vi "Periodic Tasks.vi"(8 "error in":errorcluster) -> ()   [LabVIEW 2014]
doc: "This VI runs in parallel to other tasks. It can contain as many user-defined periodic loops as you need. These can carry out PID or other sorts of timed response."
uses:
  <vilib>/Rock Robotics/WPI/Solenoid/WPI_SolenoidValue.ctl
  <vilib>/Rock Robotics/WPI/Joystick/WPI_JoystickGetSetRefNum.vi
  <vilib>/Rock Robotics/WPI/RobotDrive/WPI_RobotDriveGetSetRefNum.vi
  <vilib>/Rock Robotics/WPI/Compressor/WPI_CompressorGetSetRefNum.vi
  <vilib>/Rock Robotics/WPI/Ultrasonic/WPI_SonarMB1010DigitalRefNum Registry Get.vi
  Robot Global Data.vi
  <vilib>/Rock Robotics/Network Tables/SD Write Number.vi
  <vilib>/Rock Robotics/WPI/Ultrasonic/WPI_SonarMB1010DigitalGetRange.vi
  <vilib>/Rock Robotics/Network Tables/SD Read Boolean.vi
  <vilib>/Rock Robotics/Network Tables/SD Write Boolean.vi
  <vilib>/Rock Robotics/WPI/Solenoid/WPI_SolenoidSetEnum.vi
  <vilib>/Rock Robotics/Network Tables/SD Write Numeric Array.vi
  <vilib>/addons/control/pid/pid.llb/PID (DBL).vi
  <vilib>/Rock Robotics/Network Tables/SD Write Boolean Array.vi
  <vilib>/addons/control/pid/NI_PID_pid.lvlib
panel:
  in  "Sonar Limit":dbl
  in  "Sonar Offset":dbl
  out "Sonar Distance":dbl=36.82278911564626
  in  "Bypass INI Setting":bool
  in  "step inches":dbl=0.5
  out "Compressor Running":bool
  out "Enabled":bool=TRUE
  out "Manual Winch 2":bool
  in  "Manul drive offset 2":dbl
  in  "Manual scale 2":dbl=2.0 format="%#_13g"
  out "MV: 2":dbl(slide)=2.092346938775512 scale=-100.0..100.0
  out "PV: 2":dbl(slide)=26.0 scale=0.0..100.0
  in  "PID gains 2":T1={"proportional gain (Kc)"=0.6, "integral time (Ti, min)"=0.0, "derivative time (Td, min)"=0.0} {"derivative time (Td, min)" format="%.3f"; "integral time (Ti, min)" format="%.3f"; "proportional gain (Kc)" format="%.3f"}
  in  "output range 2":cluster{"output high":dbl, "output low":dbl}={"output high"=100.0, "output low"=-100.0} {"output low" format="%.2f"; "output high" format="%.2f"}
  out "Process variable and Setpoint 2":cluster{"initial PV":dbl, "SP:":dbl}(graph)={"initial PV"=22.512755102040813, "SP:"=26.0}
  in  "Reset Encoder? 2":bool
  out "Encoder Direction 2":string="Down"
  out "Encoder Distance 2":dbl=22.512755102040813
  in  "Encoder 2 scale":dbl=19.6
  out "In Range? 2":bool=TRUE
  in  "lower limit 2":dbl
  in  "upper limit 2":dbl=100.0
  in  "step inches 2":dbl=0.5
  out "Process variable and Setpoint":cluster{"initial PV":dbl, "SP:":dbl}(graph)={"initial PV"=107.51666666666667, "SP:"=110.0}
  in  "PID gains":T1={"proportional gain (Kc)"=1.0, "integral time (Ti, min)"=0.0, "derivative time (Td, min)"=0.0} {"derivative time (Td, min)" format="%.3f"; "integral time (Ti, min)" format="%.3f"; "proportional gain (Kc)" format="%.3f"}
  out "PV:":dbl(slide)=107.51666666666667 scale=0.0..75.0
  out "SP:":dbl(slide)=110.0 min=0.0 max=0.0 scale=0.0..75.0
  out "MV:":dbl(slide)=2.4833333333333343 scale=-100.0..100.0
  in  "output range":cluster{"output high":dbl, "output low":dbl}={"output high"=5.0, "output low"=-5.0} {"output low" format="%.2f"; "output high" format="%.2f"}
  out "In Range?":bool
  in  "lower limit":dbl
  in  "upper limit":dbl=100.0
  in  "Reset Encoder?":bool
  out "Encoder Direction":string="Down"
  out "Encoder Distance":dbl=107.51666666666667
  in  "Encoder 1 scale":dbl=30.0
  out "Manual Winch 1":bool
  in  "Manul drive offset":dbl
  in  "Manual scale 1":dbl=50.0 format="%#_13g"
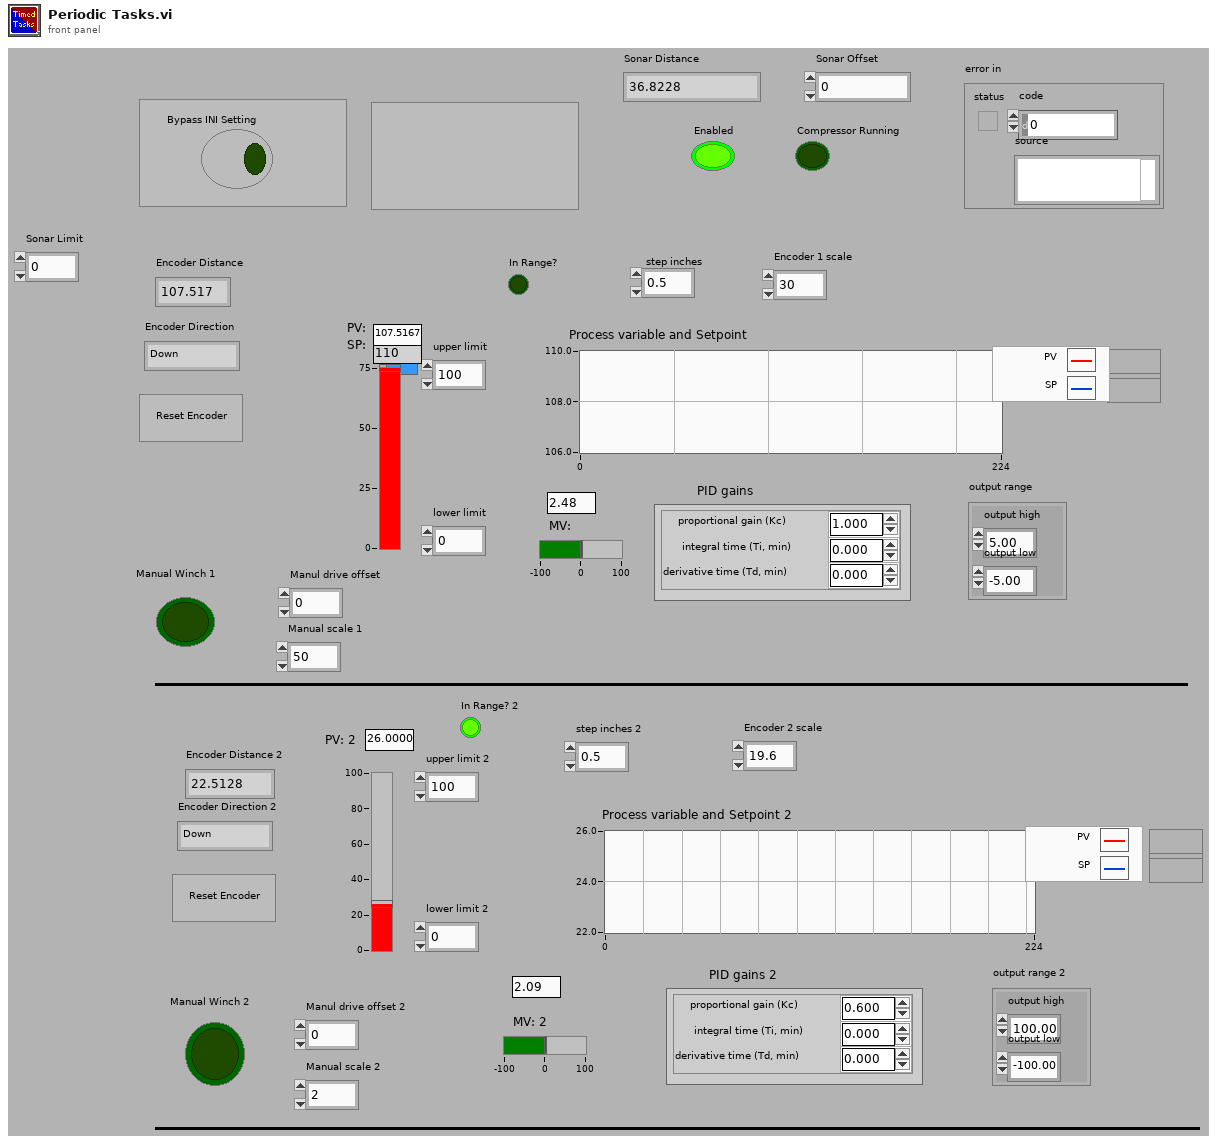
[diagram p1: front panel]
types:
  T1 = cluster{"proportional gain (Kc)":dbl, "integral time (Ti, min)":dbl, "derivative time (Td, min)":dbl}
  T2 = typedef "WPI_MotorControlDeviceRef.ctl" = cluster{"DeviceStatus":errorcluster, "Type":T3, "PWM":cluster{"Controller":T4, "PWM Channel":T5, "DeadBand":T6}, "CAN":cluster{"Device Number":u8, "Control Mode":T7, "Semaphore":T8, "Max Vout":dbl, "TalonSRX Control Mode":T9}, "Invert":bool, "TransformRef":T10, "InvTransformRef":T10}
  T3 = typedef "WPI_MotorControlType.ctl" = enum16{"PWM", "CAN", "CANTalonSRX"}
  T4 = typedef "FPGA_TypedefDigitalModule.ctl" = enum16{"Controller 1"}
  T5 = typedef "FPGA_DIOPWMChannel.ctl" = enum8{"PWM 0", "PWM 1", "PWM 2", "PWM 3", "PWM 4", "PWM 5", "PWM 6", "PWM 7", "PWM 8", "PWM 9", "PWM MXP 0", "PWM MXP 1", "PWM MXP 2", "PWM MXP 3", "PWM MXP 4", "PWM MXP 5", "PWM MXP 6", "PWM MXP 7", "PWM MXP 8", "PWM MXP 9", "Invalid"}
  T6 = typedef "WPI_PWMDeadband.ctl" = cluster{"Name":string, "maxPositivePwm":i32, "minPositivePwm":i32, "centerPwm":i32, "maxNegativePwm":i32, "minNegativePwm":i32, "angularRange":u16}
  T7 = typedef "WPI_CANJaguar_ControlMode.ctl" = enum8{"Percent VBus", "Current", "Speed", "Position", "Voltage"}
  T8 = typedef "Semaphore RefNum" = refnum<k1>
  T9 = typedef "WPI_CANTalonSRX_APIControlMode.ctl" = enum8{"Percent VBus", "Speed", "Position", "Slave", "Unchanged / Invalid"}
  T10 = typedef "WPI_PWMTransform_ConPane.ctl" = refnum<vi>
  T11 = typedef "WPI_JoystickDevRef.ctl" = cluster{"Device":T12}
  T12 = typedef "WPI_JoystickDeviceEnum.ctl" = enum16{"USB 0", "USB 1", "USB 2", "USB 3", "USB 4", "USB 5"}
  T13 = typedef "WPI_RobotDriveDevRef.ctl" = cluster{"DevStatus":errorcluster, "Motors[]":T2[], "Square Inputs":bool, "Max Output":dbl}
  T14 = typedef "WPI_CompressorDevRef.ctl" = cluster{"DevStatus":errorcluster, "Pneumatics Control Module":u8}
  T15 = typedef "WPI_SonarMB1010DigitalDeviceRef.ctl" = cluster{"CounterDevRef":T16, "Scaling factor (s/in)":dbl}
  T16 = typedef "WPI_CounterDevRef.ctl" = cluster{"DevStatus":errorcluster, "CntIndex":T17}
  T17 = typedef "FPGA_CounterCtrSystemIndex.ctl" = enum8{"Ctr 0", "Ctr 1", "Ctr 2", "Ctr 3", "Ctr 4", "Ctr 5", "Ctr 6", "Ctr 7", "Invalid"}
  T18 = typedef "WPI_SwitchDevRef.ctl" = cluster{"DevStatus":errorcluster, "DIO Channel":T19, "Controller":T4, "CntIndex":T17, "Normally Closed":bool}
  T19 = typedef "FPGA_DIOChannel.ctl" = enum8{"DIO 0", "DIO 1", "DIO 2", "DIO 3", "DIO 4", "DIO 5", "DIO 6", "DIO 7", "DIO 8", "DIO 9", "DIO MXP 0", "DIO MXP 1", "DIO MXP 2", "DIO MXP 3", "DIO MXP 4", "DIO MXP 5", "DIO MXP 6", "DIO MXP 7", "DIO MXP 8", "DIO MXP 9", "DIO MXP 10", "DIO MXP 11", "DIO MXP 12", "DIO MXP 13", "DIO MXP 14", "DIO MXP 15", "Invalid"}
  T20 = cluster{"JoystickDevRef":T11, "RobotDriveDevRef":T13}
  T21 = typedef "WPI_EncoderDevRef.ctl" = cluster{"DevStatus":errorcluster, "EncoderIndex":T22, "CounterIndex":T17, "DistancePerCount":dbl, "Decoding Type":T23}
  T22 = typedef "FPGA_EncoderIdx.ctl" = enum8{"Enc 0", "Enc 1", "Enc 2", "Enc 3", "Enc 4", "Enc 5", "Enc 6", "Enc 7", "Invalid"}
  T23 = typedef "WPI_EncoderType.ctl" = enum16{"1x", "2x", "4x"}
  T24 = typedef "WPI_SolenoidDevRef.ctl" = cluster{"DevStatus":errorcluster, "Pneumatics Control Module":u8, "Forward Solenoid Channel":T25, "Reverse Solenoid Channel":T25}
  T25 = typedef "WPI_SolenoidChannel.ctl" = enum8{"Solenoid 0", "Solenoid 1", "Solenoid 2", "Solenoid 3", "Solenoid 4", "Solenoid 5", "Solenoid 6", "Solenoid 7", "Invalid"}
  T26 = typedef "WPI_SolenoidValue.ctl" = enum16{"Off", "On", "Forward", "Reverse"}
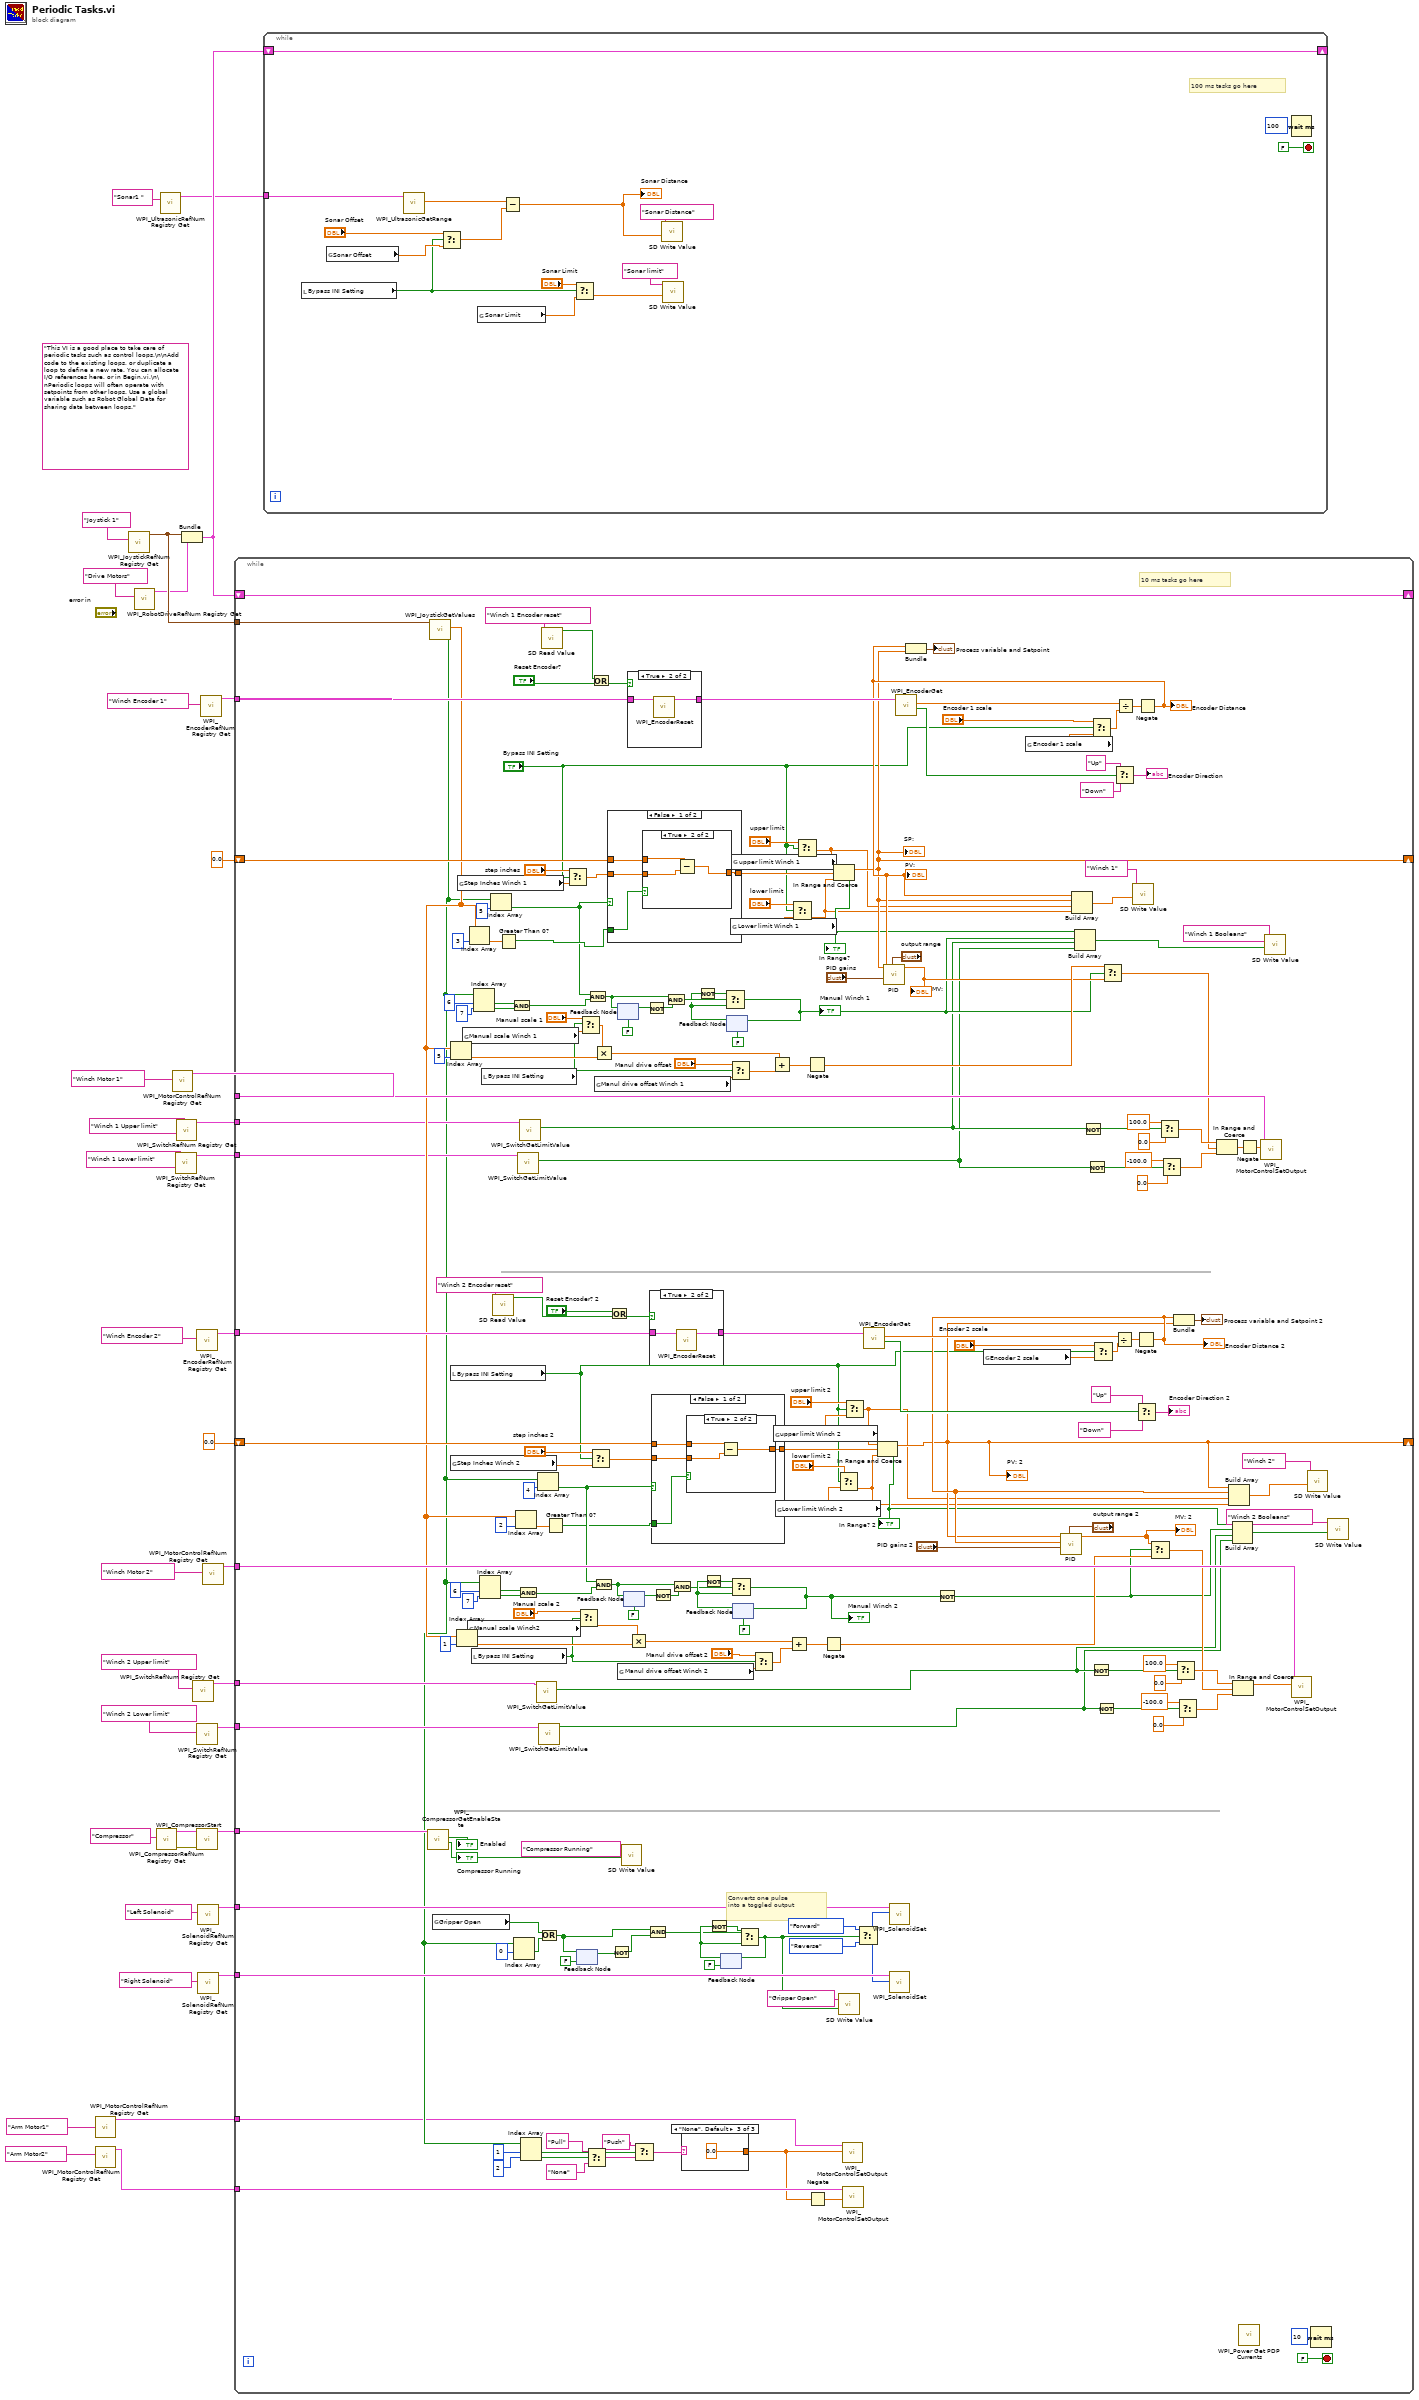
[diagram p0: block diagram]
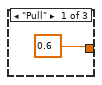
[diagram p2: hidden frame]
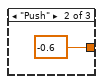
[diagram p3: hidden frame]
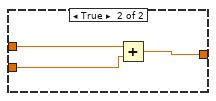
[diagram p6: hidden frame]
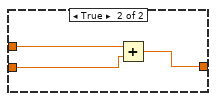
[diagram p9: hidden frame]
diagram:
  (unwired) "This VI is a good place to take care of periodic tasks such as control loops.\n\nAdd code to the existing loops, or duplicate a loop to define a new rate. You can allocate I/O references here, or in Begin.vi.\n\nPeriodic loops will often operate with setpoints from other loops. Use a global variable such as Robot Global Data for sharing data between loops."
  n1 = call <vilib>:"WPI_MotorControlRefNum Registry Get.vi"("refnum name"="Arm Motor1") -> ("MotorControlDevRef"=w2:T2)  [unwired: 9 in, 1 out]
  n2 = call <vilib>:"WPI_MotorControlRefNum Registry Get.vi"("refnum name"="Arm Motor2") -> ("MotorControlDevRef"=w1:T2)  [unwired: 9 in, 1 out]
  n3 = call <vilib>:"WPI_JoystickRefNum Registry Get.vi"("refnum name"="Joystick 1") -> ("JoystickDevRef"=w36:T11)  [unwired: 1 in, 9 out]
  n4 = call <vilib>:"WPI_RobotDriveRefNum Registry Get.vi"("refnum name"="Drive Motors") -> ("RobotDriveDevRef"=w30:T13)  [unwired: 1 in, 9 out]
  n5 = call <vilib>:"WPI_CompressorRefNum Registry Get.vi"("refnum name"="Compressor") -> ("error out"=w14:errorcluster, "CompressorDevRef"=w13:T14)  [unwired: 9 in]
  n6 = call-poly <vilib>:"WPI_UltrasonicRefNum Registry Get.vi"("refnum name"="Sonar1 ") -> ("SonarMB1010DigitalDevRef"=w5:T15)  [unwired: 9 in, 1 out]
  n7 = call <vilib>:"WPI_MotorControlRefNum Registry Get.vi"("refnum name"="Winch Motor 1") -> ("MotorControlDevRef"=w35:T2)  [unwired: 9 in, 1 out]
  n8 = call <vilib>:"WPI_SwitchRefNum Registry Get.vi"("refnum name"="Winch 1 Lower limit") -> ("SwitchDevRef"=w21:T18)  [unwired: 9 in, 1 out]
  n9 = call <vilib>:"WPI_SwitchRefNum Registry Get.vi"("refnum name"="Winch 1 Upper limit") -> ("SwitchDevRef"=w20:T18)  [unwired: 9 in, 1 out]
  n10 = Bundle("JoystickDevRef"=w36, "RobotDriveDevRef"=w30) -> (w31:T20)  [unwired: 1 out]
  n11 = call <vilib>:"WPI_SwitchRefNum Registry Get.vi"("refnum name"="Winch 2 Upper limit") -> ("SwitchDevRef"=w19:T18)  [unwired: 9 in, 1 out]
  n12 = call <vilib>:"WPI_CompressorStart.vi"("error in (no error)"=w14, "CompressorDevRef"=w13) -> ("CompressorDevRef"=w11:T14)  [unwired: 8 in, 1 out]
  n13 = call <vilib>:"WPI_EncoderRefNum Registry Get.vi"("refnum name"="Winch Encoder 2") -> ("EncoderDevRef"=w24:T21)  [unwired: 9 in, 1 out]
  n14 = call <vilib>:"WPI_SwitchRefNum Registry Get.vi"("refnum name"="Winch 2 Lower limit") -> ("SwitchDevRef"=w18:T18)  [unwired: 9 in, 1 out]
  n15 = call <vilib>:"WPI_SolenoidRefNum Registry Get.vi"("refnum name"="Left Solenoid") -> ("SolenoidDevRef"=w8:T24)  [unwired: 9 in, 1 out]
  n16 = call <vilib>:"WPI_SolenoidRefNum Registry Get.vi"("refnum name"="Right Solenoid") -> ("SolenoidDevRef"=w7:T24)  [unwired: 9 in, 1 out]
  n17 = call <vilib>:"WPI_EncoderRefNum Registry Get.vi"("refnum name"="Winch Encoder 1") -> ("EncoderDevRef"=w32:T21)  [unwired: 9 in, 1 out]
  n18 = call <vilib>:"WPI_MotorControlRefNum Registry Get.vi"("refnum name"="Winch Motor 2") -> ("MotorControlDevRef"=w26:T2)  [unwired: 9 in, 1 out]
  n19 = while {
    shift-right: [w230] -> _
    shift-left: w31 -> [w230]
    tunnel: w32 -> [w234]
    shift-right: [w134] -> _
    shift-left: 0.0 ("upper limit") -> [w233]
    tunnel: w35 -> [w231]
    tunnel: w36 -> [w229]
    shift-right: [w117] -> _
    shift-left: 0.0 ("upper limit") -> [w204]
    tunnel: w26 -> [w202]
    tunnel: w24 -> [w194]
    tunnel: w21 -> [w171]
    tunnel: w20 -> [w170]
    tunnel: w18 -> [w157]
    tunnel: w19 -> [w158]
    tunnel: w11 -> [w148]
    tunnel: w8 -> [w146]
    tunnel: w7 -> [w143]
    tunnel: w2 -> [w43]
    tunnel: w1 -> [w42]
    stop <- FALSE stop-if-true
    # "Converts one pulse\ninto a toggled output"
    # "10 ms tasks go here"
    n20 = call <vilib>:"WPI_CompressorGetEnableState.vi"("CompressorDevRef"=w148) -> ("Compressor Running"=w68:bool, "Enabled"=→"Enabled":bool)  [unwired: 7 in, 2 out]
    "Compressor Running" <- w68
    n21 = call <vilib>:"WPI_JoystickGetValues.vi"("JoystickDevRef"=w229) -> ("Buttons"=w51:bool[], "Axes"=w172:dbl[])  [unwired: 6 in, 3 out]
    n22 = global read "Robot Global Data.vi" "Gripper Open"() -> (w145:bool)
    n23 = Index Array(array=w172, index=5) -> (element=w211:dbl)
    n24 = local read "Bypass INI Setting"() -> (w78:bool)
    n25 = global read "Robot Global Data.vi" "Step Inches Winch 2"() -> (w83:dbl)
    n26 = Index Array(array=w172, index=1) -> (element=w190:dbl)
    n27 = global read "Robot Global Data.vi" "Step Inches Winch 1"() -> (w97:dbl)
    n28 = global read "Robot Global Data.vi" "Manual scale Winch 1"() -> (w92:dbl)
    n29 = global read "Robot Global Data.vi" "Manual scale Winch2"() -> (w74:dbl)
    n30 = Index Array(array=w172, index=3) -> (element=w228:dbl)
    n31 = local read "Bypass INI Setting"() -> (w71:bool)
    n32 = Index Array(array=w51, index #1=6 ("index"), index #2=7 ("index")) -> (element #1=w223:bool, element #2=w224:bool)
    n33 = Index Array(array=w51, index #1=6 ("index"), index #2=7 ("index")) -> (element #1=w178:bool, element #2=w177:bool)
    n34 = local read "Bypass INI Setting"() -> (w90:bool)
    n35 = Index Array(array=w51, index=5) -> (element=w52:bool)
    n36 = call-poly <vilib>:"SD Read Value.vi"("Name"="Winch 2 Encoder reset") -> ("Boolean"=w108:bool)  [unwired: 8 in, 2 out]
    n37 = Greater Than 0?(x=w228) -> (x > 0?=w53:bool)
    n38 = And(x=w223, y=w224) -> (x .and. y?=w222:bool)
    n39 = Index Array(array=w51, index #1=0 ("index")) -> (element #1=w142:bool)  [unwired: 1 in, 1 out]
    n40 = Index Array(array=w172, index=2) -> (element=w208:dbl)
    n41 = call <vilib>:"WPI_SwitchGetLimitValue.vi"("SwitchDevRef"=w171) -> ("Switch Pressed"=w124:bool)  [unwired: 8 in, 2 out]
    n42 = And(x=w178, y=w177) -> (x .and. y?=w179:bool)
    n43 = call <vilib>:"WPI_SwitchGetLimitValue.vi"("SwitchDevRef"=w170) -> ("Switch Pressed"=w125:bool)  [unwired: 8 in, 2 out]
    n44 = Index Array(array=w51, index #1=1, index #2=2) -> (element #1=w50:bool, element #2=w49:bool)
    n45 = call <vilib>:"WPI_SwitchGetLimitValue.vi"("SwitchDevRef"=w158) -> ("Switch Pressed"=w113:bool)  [unwired: 8 in, 2 out]
    n46 = Index Array(array=w51, index=4) -> (element=w57:bool)
    n47 = call <vilib>:"WPI_SwitchGetLimitValue.vi"("SwitchDevRef"=w157) -> ("Switch Pressed"=w112:bool)  [unwired: 8 in, 2 out]
    n48 = Or(x=w145, y=w142) -> (x .or. y?=w63:bool)
    n49 = call-poly <vilib>:"SD Read Value.vi"("Name"="Winch 1 Encoder reset") -> ("Boolean"=w127:bool)  [unwired: 8 in, 2 out]
    n50 = Greater Than 0?(x=w208) -> (x > 0?=w56:bool)
    n51 = Select(t="step inches", s="Bypass INI Setting", f=w97) -> (s? t:f=w99:dbl)
    n52 = feedback #1(FALSE ("Button 1")) -> (w66:bool)
    n53 = feedback-in #1(w63) -> ()
    n54 = Select(t="Manual scale 2", s=w71, f=w74) -> (s? t:f=w76:dbl)
    n55 = Select(t="Manual scale 1", s=w90, f=w92) -> (s? t:f=w94:dbl)
    n56 = Select(t="Pull", s=w49, f="None") -> (s? t:f=w48:string)
    n57 = And(x=w52, y=w222) -> (x .and. y?=w221:bool)
    n58 = Select(t="step inches 2", s=w78, f=w83) -> (s? t:f=w84:dbl)
    n59 = Or(x=w127, y="Reset Encoder?") -> (x .or. y?=w128:bool)
    n60 = Multiply(x=w94, y=w211) -> (x*y=w95:dbl)
    n61 = And(x=w57, y=w179) -> (x .and. y?=w180:bool)
    n62 = global read "Robot Global Data.vi" "Manul drive offset Winch 1"() -> (w89:dbl)
    n63 = case shown="False" w52 {
      tunnel: w233 -> [w272 w279]
      tunnel: [w271 w278] -> w243
      tunnel: w99 -> [w270 w277]
      tunnel: w53 -> [w269 _]
      frame False {
        n64 = case shown="True" w269 {
          tunnel: [w273 w276] -> w271
          tunnel: w272 -> [w273 w275]
          tunnel: w270 -> [_ w274]
          frame False {
          }
          frame True {
            n65 = Subtract(x=w275, y=w274) -> (x-y=w276:dbl)
          }
        }
      }
      frame True {
        n66 = Add(x=w279, y=w277) -> (x+y=w278:dbl)
      }
    }
    n67 = Or(x="Reset Encoder? 2", y=w108) -> (x .or. y?=w110:bool)
    n68 = Not(x=w66) -> (.not. x?=w65:bool)
    n69 = feedback #2(FALSE) -> (w219:bool)
    n70 = feedback-in #2(w221) -> ()
    n71 = global read "Robot Global Data.vi" "Manul drive offset Winch 2"() -> (w70:dbl)
    n72 = call-poly <vilib>:"SD Write Value.vi"("Boolean"=w68, "Name"="Compressor Running") -> ()  [unwired: 8 in, 2 out]
    n73 = feedback #3(FALSE) -> (w182:bool)
    n74 = feedback-in #3(w180) -> ()
    n75 = case shown="True" w128 {
      tunnel: w234 -> [w266 w268]
      tunnel: [w266 w267] -> w241
      frame False {
      }
      frame True {
        n76 = call <vilib>:"WPI_EncoderReset.vi"("EncoderDevRef"=w268) -> ("EncoderDevRef"=w267:T21)  [unwired: 1 in, 9 out]
      }
    }
    n77 = Multiply(x=w76, y=w190) -> (x*y=w191:dbl)
    n78 = Select(t="Push", s=w50, f=w48) -> (s? t:f=w44:string)
    n79 = Not(x=w219) -> (.not. x?=w220:bool)
    n80 = And(x=w63, y=w65) -> (x .and. y?=w58:bool)
    n81 = case shown="True" w110 {
      tunnel: w194 -> [w252 w254]
      tunnel: [w252 w253] -> w196
      frame False {
      }
      frame True {
        n82 = call <vilib>:"WPI_EncoderReset.vi"("EncoderDevRef"=w254) -> ("EncoderDevRef"=w253:T21)  [unwired: 1 in, 9 out]
      }
    }
    n83 = case shown="False" w57 {
      tunnel: w204 -> [w258 w265]
      tunnel: [w257 w264] -> w205
      tunnel: w84 -> [w256 w263]
      tunnel: w56 -> [w255 _]
      frame False {
        n84 = case shown="True" w255 {
          tunnel: [w259 w262] -> w257
          tunnel: w258 -> [w259 w261]
          tunnel: w256 -> [_ w260]
          frame False {
          }
          frame True {
            n85 = Subtract(x=w261, y=w260) -> (x-y=w262:dbl)
          }
        }
      }
      frame True {
        n86 = Add(x=w265, y=w263) -> (x+y=w264:dbl)
      }
    }
    n87 = Not(x=w182) -> (.not. x?=w181:bool)
    n88 = And(x=w221, y=w220) -> (x .and. y?=w217:bool)
    n89 = And(x=w180, y=w181) -> (x .and. y?=w184:bool)
    n90 = case shown="\"None\", Default" w44 {
      tunnel: [0.6 -0.6 0.0] -> w41
      frame "Pull" {
      }
      frame "Push" {
      }
      frame "None", Default {
      }
    }
    n91 = feedback #4(FALSE) -> (w62:bool)
    n92 = Not(x=w62) -> (.not. x?=w61:bool)
    n93 = feedback #5(FALSE) -> (w216:bool)
    n94 = Not(x=w216) -> (.not. x?=w214:bool)
    n95 = Select(t=w214, s=w217, f=w216) -> (s? t:f=w131:bool)
    "Manual Winch 1" <- w131
    n96 = feedback-in #5(w131) -> ()
    n97 = Select(t="Manul drive offset", s=w90, f=w89) -> (s? t:f=w88:dbl)
    n98 = global read "Robot Global Data.vi" "Lower limit Winch 1"() -> (w101:dbl)
    n99 = global read "Robot Global Data.vi" "upper limit Winch 1"() -> (w100:dbl)
    n100 = feedback #6(FALSE) -> (w185:bool)
    n101 = Not(x=w185) -> (.not. x?=w187:bool)
    n102 = Select(t=w187, s=w184, f=w185) -> (s? t:f=w173:bool)
    "Manual Winch 2" <- w173
    n103 = feedback-in #6(w173) -> ()
    n104 = Select(t=w61, s=w58, f=w62) -> (s? t:f=w59:bool)
    n105 = feedback-in #4(w59) -> ()
    n106 = Select(t="Manul drive offset 2", s=w71, f=w70) -> (s? t:f=w73:dbl)
    n107 = Add(x=w95, y=w88) -> (x+y=w212:dbl)
    n108 = global read "Robot Global Data.vi" "upper limit Winch 2"() -> (w81:dbl)
    n109 = global read "Robot Global Data.vi" "Lower limit Winch 2"() -> (w77:dbl)
    n110 = Add(x=w191, y=w73) -> (x+y=w189:dbl)
    n111 = Select(t="lower limit", s="Bypass INI Setting", f=w101) -> (s? t:f=w103:dbl)
    n112 = Select(t="upper limit", s="Bypass INI Setting", f=w100) -> (s? t:f=w104:dbl)
    n113 = Negate(x=w212) -> (-x=w210:dbl)
    n114 = Negate(x=w41) -> (-x=w40:dbl)
    n115 = Negate(x=w189) -> (-x=w174:dbl)
    n116 = In Range and Coerce(upper limit=w104, x=w243, lower limit=w103) -> (coerced(x)=w134:dbl, In Range?=w132:bool)
    "SP:" <- w134
    "In Range?" <- w132
    n117 = Select(t="lower limit 2", s=w78, f=w77) -> (s? t:f=w80:dbl)
    n118 = call-poly <vilib>:"SD Write Value.vi"("Boolean"=w59, "Name"="Gripper Open") -> ()  [unwired: 8 in, 2 out]
    n119 = call <vilib>:"WPI_MotorControlSetOutput.vi"("Output"=w41, "MotorControlDevRef"=w43) -> ()  [unwired: 7 in, 3 out]
    n120 = call <vilib>:"WPI_MotorControlSetOutput.vi"("Output"=w40, "MotorControlDevRef"=w42) -> ()  [unwired: 7 in, 3 out]
    n121 = Select(t="upper limit 2", s=w78, f=w81) -> (s? t:f=w82:dbl)
    n122 = Select(t=WPI_SolenoidValue."Forward" ("Value"), s=w59, f=WPI_SolenoidValue."Reverse" ("Value")) -> (s? t:f=w137:T26)
    n123 = call <vilib>:"WPI_EncoderGet.vi"("EncoderDevRef"=w196) -> ("Direction"=w200:bool, "Distance"=w199:dbl)  [unwired: 1 in, 8 out]
    n124 = In Range and Coerce(upper limit=w82, x=w205, lower limit=w80) -> (coerced(x)=w117:dbl, In Range?=w115:bool)
    "In Range? 2" <- w115
    "PV: 2" <- w117
    n125 = call-poly <vilib>:"WPI_SolenoidSet.vi"("Value"=w137, "SolenoidDevRef"=w146) -> ()  [unwired: 8 in, 2 out]
    n126 = call-poly <vilib>:"WPI_SolenoidSet.vi"("Value"=w137, "SolenoidDevRef"=w143) -> ()  [unwired: 8 in, 2 out]
    n127 = call <vilib>:"WPI_EncoderGet.vi"("EncoderDevRef"=w241) -> ("Direction"=w235:bool, "Distance"=w236:dbl)  [unwired: 1 in, 8 out]
    n128 = Not(x=w173) -> (.not. x?=w114:bool)
    n129 = global read "Robot Global Data.vi" "Encoder 2 scale"() -> (w85:dbl)
    n130 = global read "Robot Global Data.vi" "Encoder 1 scale"() -> (w105:dbl)
    n131 = Build Array(w132, w131, w125, w124) -> (w133:bool[])
    n132 = Not(x=w125) -> (.not. x?=w151:bool)
    n133 = Not(x=w124) -> (.not. x?=w150:bool)
    n134 = Not(x=w113) -> (.not. x?=w156:bool)
    n135 = Select(t="Encoder 1 scale", s="Bypass INI Setting", f=w105) -> (s? t:f=w107:dbl)
    n136 = Select(t="Encoder 2 scale", s=w78, f=w85) -> (s? t:f=w87:dbl)
    n137 = Not(x=w112) -> (.not. x?=w155:bool)
    n138 = Select(t="Up", s=w235, f="Down") -> (s? t:f=→"Encoder Direction":string)
    n139 = Divide(x=w199, y=w87) -> (x/y=w201:dbl)
    n140 = Divide(x=w236, y=w107) -> (x/y=w232:dbl)
    n141 = Negate(x=w201) -> (-x=w118:dbl)
    "Encoder Distance 2" <- w118
    n142 = call-poly <vilib>:"PID.vi"("output range"="output range 2", "PID gains"="PID gains 2", "process variable"=w118, "setpoint"=w117) -> ("output"=w141:dbl)  [unwired: 6 in, 1 out]
    "MV: 2" <- w141
    n143 = Select(t="Up", s=w200, f="Down") -> (s? t:f=→"Encoder Direction 2":string)
    n144 = Negate(x=w232) -> (-x=w135:dbl)
    "PV:" <- w135
    "Encoder Distance" <- w135
    n145 = call-poly <vilib>:"PID.vi"("output range"="output range", "PID gains"="PID gains", "process variable"=w135, "setpoint"=w134) -> ("output"=w209:dbl)  [unwired: 6 in, 1 out]
    "MV:" <- w209
    n146 = Bundle(w135, "upper limit Winch 1"=w134) -> (→"Process variable and Setpoint":cluster{dbl, "upper limit Winch 1":dbl})  [unwired: 1 in]
    n147 = Build Array(w135, w134, w104, w103) -> (w136:dbl[])
    n148 = Select(t=w210, s=w131, f=w209) -> (s? t:f=w149:dbl)
    n149 = call-poly <vilib>:"SD Write Value.vi"("Numeric Array"=w136, "Name"="Winch 1") -> ()  [unwired: 8 in, 2 out]
    n150 = Select(t=w141, s=w114, f=w174) -> (s? t:f=w140:dbl)
    n151 = Select(t=100.0, s=w151, f=0.0) -> (s? t:f=w167:dbl)
    n152 = Select(t=-100.0, s=w150, f=0.0) -> (s? t:f=w168:dbl)
    n153 = Bundle(w118, "upper limit Winch 2"=w117) -> (→"Process variable and Setpoint 2":cluster{dbl, "upper limit Winch 2":dbl})  [unwired: 1 in]
    n154 = Select(t=100.0, s=w156, f=0.0) -> (s? t:f=w160:dbl)
    n155 = Select(t=-100.0, s=w155, f=0.0) -> (s? t:f=w159:dbl)
    n156 = In Range and Coerce(upper limit=w167, x=w149, lower limit=w168) -> (coerced(x)=w169:dbl)  [unwired: 1 out]
    n157 = Build Array(w117, w118, w82, w80) -> (w119:dbl[])
    n158 = Build Array(w115, w114, w113, w112) -> (w120:bool[])
    n159 = In Range and Coerce(upper limit=w160, x=w140, lower limit=w159) -> (coerced(x)=w54:dbl)  [unwired: 1 out]
    n160 = call <vilib>:"WPI_Power Get PDP Currents.vi"() -> ()  [unwired: 13 in, 3 out]
    n161 = Negate(x=w169) -> (-x=w55:dbl)
    n162 = call <vilib>:"WPI_MotorControlSetOutput.vi"("Output"=w55, "MotorControlDevRef"=w231) -> ()  [unwired: 2 in, 8 out]
    n163 = call-poly <vilib>:"SD Write Value.vi"("Boolean Array"=w133, "Name"="Winch 1 Booleans") -> ()  [unwired: 8 in, 2 out]
    n164 = call <vilib>:"WPI_MotorControlSetOutput.vi"("Output"=w54, "MotorControlDevRef"=w202) -> ()  [unwired: 2 in, 8 out]
    n165 = call-poly <vilib>:"SD Write Value.vi"("Numeric Array"=w119, "Name"="Winch 2") -> ()  [unwired: 8 in, 2 out]
    n166 = Wait (ms)(milliseconds to wait=u32 10) -> ()  [unwired: 1 out]
    n167 = call-poly <vilib>:"SD Write Value.vi"("Boolean Array"=w120, "Name"="Winch 2 Booleans") -> ()  [unwired: 8 in, 2 out]
  }
  n168 = while {
    shift-right: [w292] -> _
    shift-left: w31 -> [w292]
    tunnel: w5 -> [w290]
    stop <- FALSE stop-if-true
    # "100 ms tasks go here"
    n169 = local read "Bypass INI Setting"() -> (w280:bool)
    n170 = global read "Robot Global Data.vi" "Sonar Offset"() -> (w281:dbl)
    n171 = call-poly <vilib>:"WPI_UltrasonicGetRange.vi"("SonarMB1010DigitalDevRef"=w290) -> ("Distance"=w288:dbl)  [unwired: 8 in, 2 out]
    n172 = Select(t="Sonar Offset", s=w280, f=w281) -> (s? t:f=w283:dbl)
    n173 = global read "Robot Global Data.vi" "Sonar Limit"() -> (w286:dbl)
    n174 = Subtract(x=w288, y=w283) -> (x-y=w289:dbl)
    "Sonar Distance" <- w289
    n175 = Select(t="Sonar Limit", s=w280, f=w286) -> (s? t:f=w285:dbl)
    n176 = call-poly <vilib>:"SD Write Value.vi"("Numeric"=w289, "Name"="Sonar Distance") -> ()  [unwired: 8 in, 2 out]
    n177 = call-poly <vilib>:"SD Write Value.vi"("Numeric"=w285, "Name"="Sonar limit") -> ()  [unwired: 8 in, 2 out]
    n178 = Wait (ms)(milliseconds to wait=u32 100) -> ()  [unwired: 1 out]
  }
